vi "Secuencia.vi"(5 "Bool":bool, 8 "Estado Actual":i32, 9 "Selector Tipo":bool) -> (2 "Siguiente Estado":i32=4)   [LabVIEW 2018]
panel:
  out "Const. Sec":i32[](array[numeric])=[0, 3]
  out "AFM Sec":i32[](array[numeric])=[0, 4, 1, 5, 2, 3]
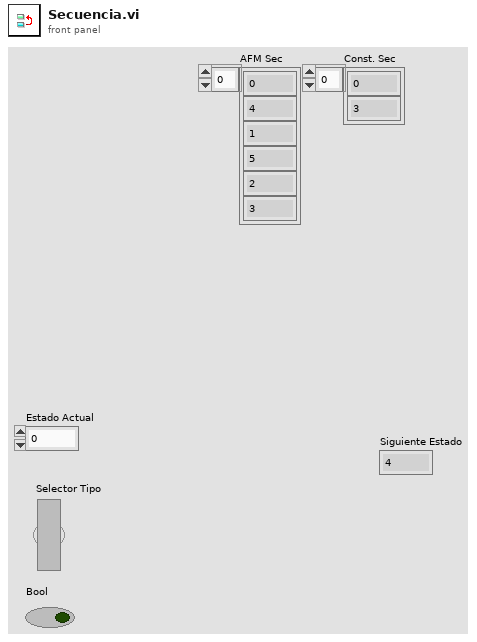
[diagram p1: front panel]
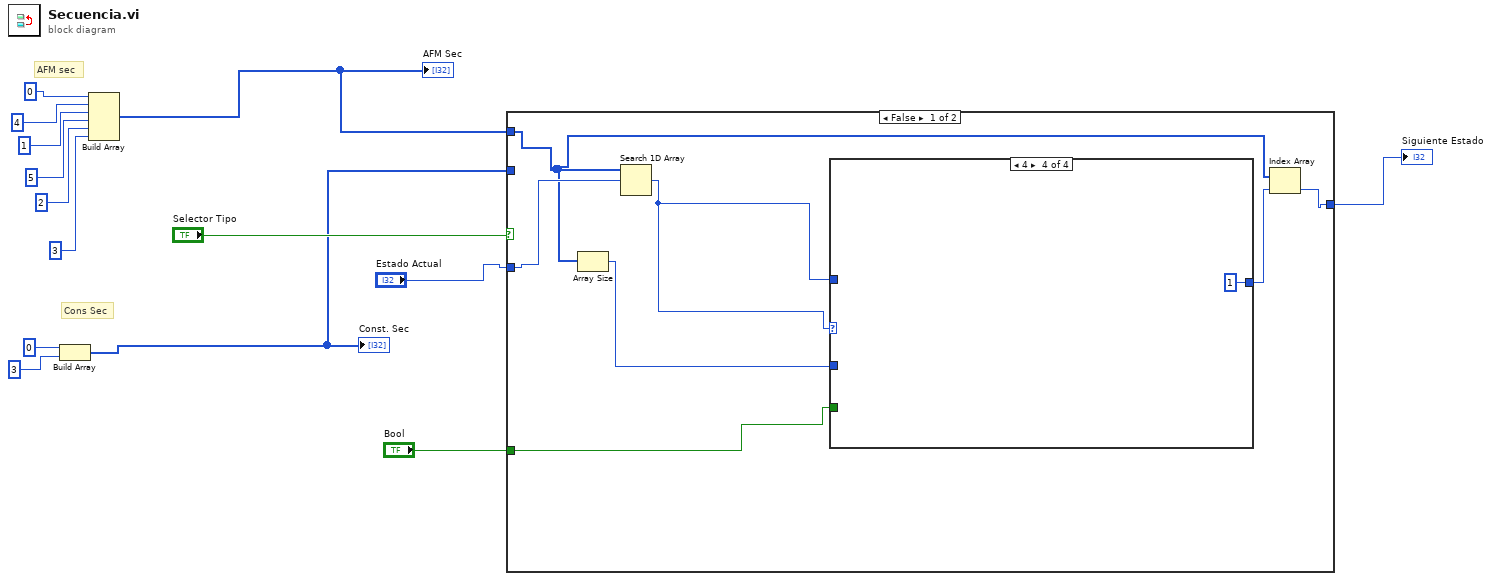
[diagram p0: block diagram]
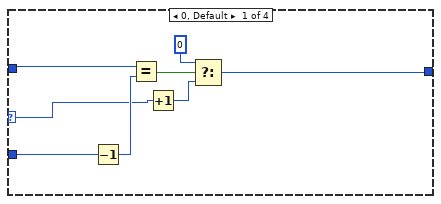
[diagram p2: hidden frame]
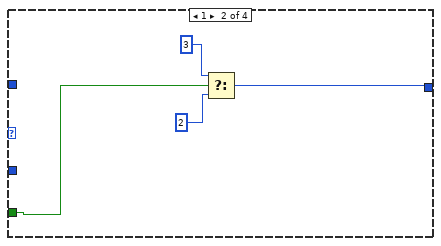
[diagram p3: hidden frame]
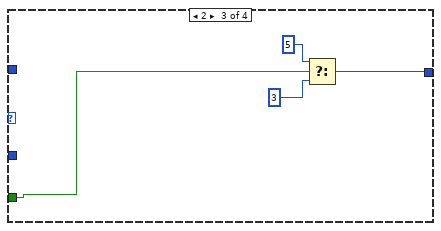
[diagram p4: hidden frame]
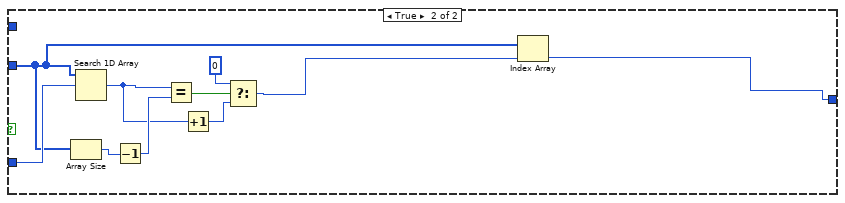
[diagram p5: hidden frame]
diagram:
  # "Cons Sec"
  # "AFM sec"
  n1 = Build Array(0, 3 ("element")) -> (w5:i32[])
  "Const. Sec" <- w5
  n2 = Build Array(0, 4 ("element"), 1 ("element"), 5 ("element"), 2 ("element"), 3 ("element")) -> (w4:i32[])
  "AFM Sec" <- w4
  n3 = case shown="False" "Selector Tipo" {
    tunnel: w5 -> [_ w41]
    tunnel: w4 -> [w17 _]
    tunnel: "Estado Actual" -> [w21 w48]
    tunnel: [w15 w39] -> w2
    tunnel: "Bool" -> [w18 _]
    frame False {
      n4 = Array Size(array=w17) -> (size(s)=w20:i32)
      n5 = Search 1D Array(1D array=w17, element=w21) -> (index of element=w19:i32)  [unwired: 1 in]
      n6 = case shown="4" w19 {
        selector: w19 -> [w23 _ _ _]
        tunnel: w20 -> [w26 _ _ _]
        tunnel: w19 -> [w24 _ _ _]
        tunnel: [w22 w33 w37 1 ("f")] -> w16
        tunnel: w18 -> [_ w31 w34 _]
        frame 0, Default {
          n7 = Decrement(x=w26) -> (x-1=w29:i32)
          n8 = Equal?(x=w24, y=w29) -> (x = y?=w27:bool)
          n9 = Increment(x=w23) -> (x+1=w28:i32)
          n10 = Select(t=0, s=w27, f=w28) -> (s? t:f=w22:i32)
        }
        frame 1 {
          n11 = Select(t=3, s=w31, f=2) -> (s? t:f=w33:i32)
        }
        frame 2 {
          n12 = Select(t=5, s=w34, f=3) -> (s? t:f=w37:i32)
        }
        frame 4 {
        }
      }
      n13 = Index Array(array=w17, index=w16) -> (element=w15:i32)
    }
    frame True {
      n14 = Array Size(array=w41) -> (size(s)=w47:i32)
      n15 = Search 1D Array(1D array=w41, element=w48) -> (index of element=w43:i32)  [unwired: 1 in]
      n16 = Decrement(x=w47) -> (x-1=w46:i32)
      n17 = Equal?(x=w43, y=w46) -> (x = y?=w45:bool)
      n18 = Increment(x=w43) -> (x+1=w42:i32)
      n19 = Select(t=0, s=w45, f=w42) -> (s? t:f=w40:i32)
      n20 = Index Array(array=w41, index=w40) -> (element=w39:i32)
    }
  }
  "Siguiente Estado" <- w2
